vi "TriggerModuloLCMultiple.vi"(11 "TriggerModulos":i32[](array[numeric])) -> (3 "LeastCommonMult":i64)   [LabVIEW 2009, in "POLARIS BME DG.lvlib"]
uses:
  POLARIS BME DG.lvlib
  <vilib>/gmath/NI_Gmath.lvlib
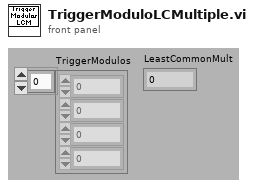
[diagram p1: front panel]
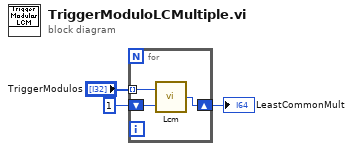
[diagram p0: block diagram]
diagram:
  n1 = for {
    tunnel: "TriggerModulos" -> [w5] mode=indexing
    shift-right: [w6] -> w3
    shift-left: 1 ("lcm(x,y)") -> [w4]
    n2 = call <vilib>:"Lcm.vi"("y"=w4, "x"=w5) -> ("lcm(x,y)"=w6:i32)
  }
  "LeastCommonMult" <- w3
